vi "testCreateNotifierStopServer.vi"(8 "error in (no error)":errorcluster) -> (0 "error out":errorcluster)   [LabVIEW 2018]
uses:
  src/TcpServerBase/TcpServerBase.lvclass
  <vilib>/addons/_JKI Toolkits/Caraya/classes/Assert/Assert Equal Type_Variant.vi
  <vilib>/addons/_JKI Toolkits/Caraya/classes/Test/Test.lvclass
  <vilib>/addons/_JKI Toolkits/Caraya/classes/Assert/Assert.lvclass
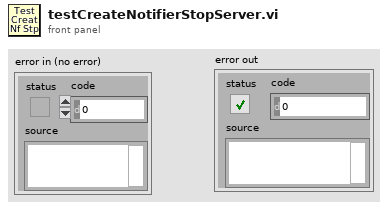
[diagram p1: front panel]
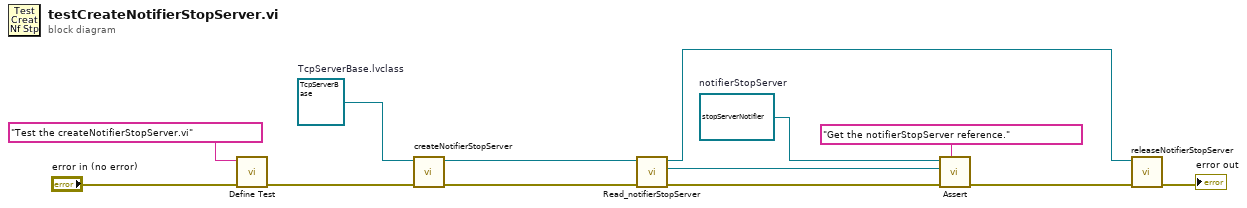
[diagram p0: block diagram]
diagram:
  w3 = refnum<notifier> refnum  # notifierStopServer
  w9 = refnum<class "TcpServerBase.lvclass"> refnum  # TcpServerBase.lvclass
  n1 = call <vilib>:"Define Test.vi"("error in (no error)"="error in (no error)", "Label (VI Title)"="Test the createNotifierStopServer.vi") -> ("error out"=w8:errorcluster)  [unwired: 9 in]
  n2 = call "createNotifierStopServer.vi"("error in (no error)"=w8, "tcpServerBase in"=w9) -> ("error out"=w6:errorcluster, "tcpServerBase out"=w7:refnum<class "TcpServerBase.lvclass">)  [unwired: 8 in]
  n3 = call "Read_notifierStopServer.vi"("error in (no error)"=w6, "TcpServerBase in"=w7) -> ("error out"=w5:errorcluster, "notifierStopServer"=w4:refnum<notifier>, "TcpServerBase out"=w1:refnum<class "TcpServerBase.lvclass">)  [unwired: 7 in]
  n4 = call-poly <vilib>:"Assert.vi"("Label"="Get the notifierStopServer reference.", "error in (no error)"=w5, "Y"=w4, "X"=w3) -> ("error out"=w11:errorcluster)  [unwired: 7 in]
  n5 = call "releaseNotifierStopServer.vi"("error in (no error)"=w11, "tcpServerBase in"=w1) -> ("error out"=→"error out":errorcluster)  [unwired: 8 in, 1 out]
